vi "Message References to Message Handles.vi"(8 "error in":errorcluster, 11 "message refs":T2[](array[typedef]) format="%.0x") -> (0 "error out":errorcluster, 3 "message handles":cluster{"parameters":T1[], "timestamps":T2[]} {"timestamps" format="%.0x"; "parameters"."RxBC channel handle" format="%.0x"; "parameters"."RxRT channel handle" format="%.0x"; "parameters"."Tx channel handle" format="%.0x"})   [LabVIEW 2020, in "Ballard MIL-STD-1553 Engine.lvlib" / "Implementation.lvlib" / "Execution Unit.lvclass"]
uses:
  Execution Unit.lvclass
  <vilib>/NI VeriStand/Custom Device API/Custom Device Item Ref.ctl
  <vilib>/NI VeriStand/Custom Device API/Custom Device API.lvlib
  Scripting/Ballard MIL-STD-1553 Scripting.lvlib
  Parameter Handles.ctl
  Message Handles.ctl
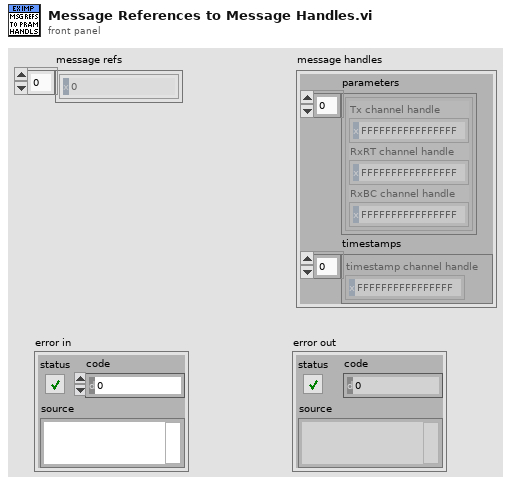
[diagram p1: front panel]
types:
  T1 = typedef "Ballard MIL-STD-1553 Engine.lvlib/Implementation.lvlib/Execution Unit.lvclass/Parameter Handles.ctl" = cluster{"Tx channel handle":T2, "RxRT channel handle":T2, "RxBC channel handle":T2}
  T2 = typedef "Custom Device API.lvlib/Custom Device Item Ref.ctl" = u64
  T3 = typedef "Ballard MIL-STD-1553 Engine.lvlib/Implementation.lvlib/Execution Unit.lvclass/Message Handles.ctl" = cluster{"parameters":T1[], "timestamps":T2[]}
  T4 = typedef "Direction.ctl" = enum16{"Rx", "Tx"}
  T5 = typedef "Terminal Endpoint.ctl" = cluster{"terminal address":T6, "subaddress":T6}
  T6 = typedef "Address.ctl" = u16
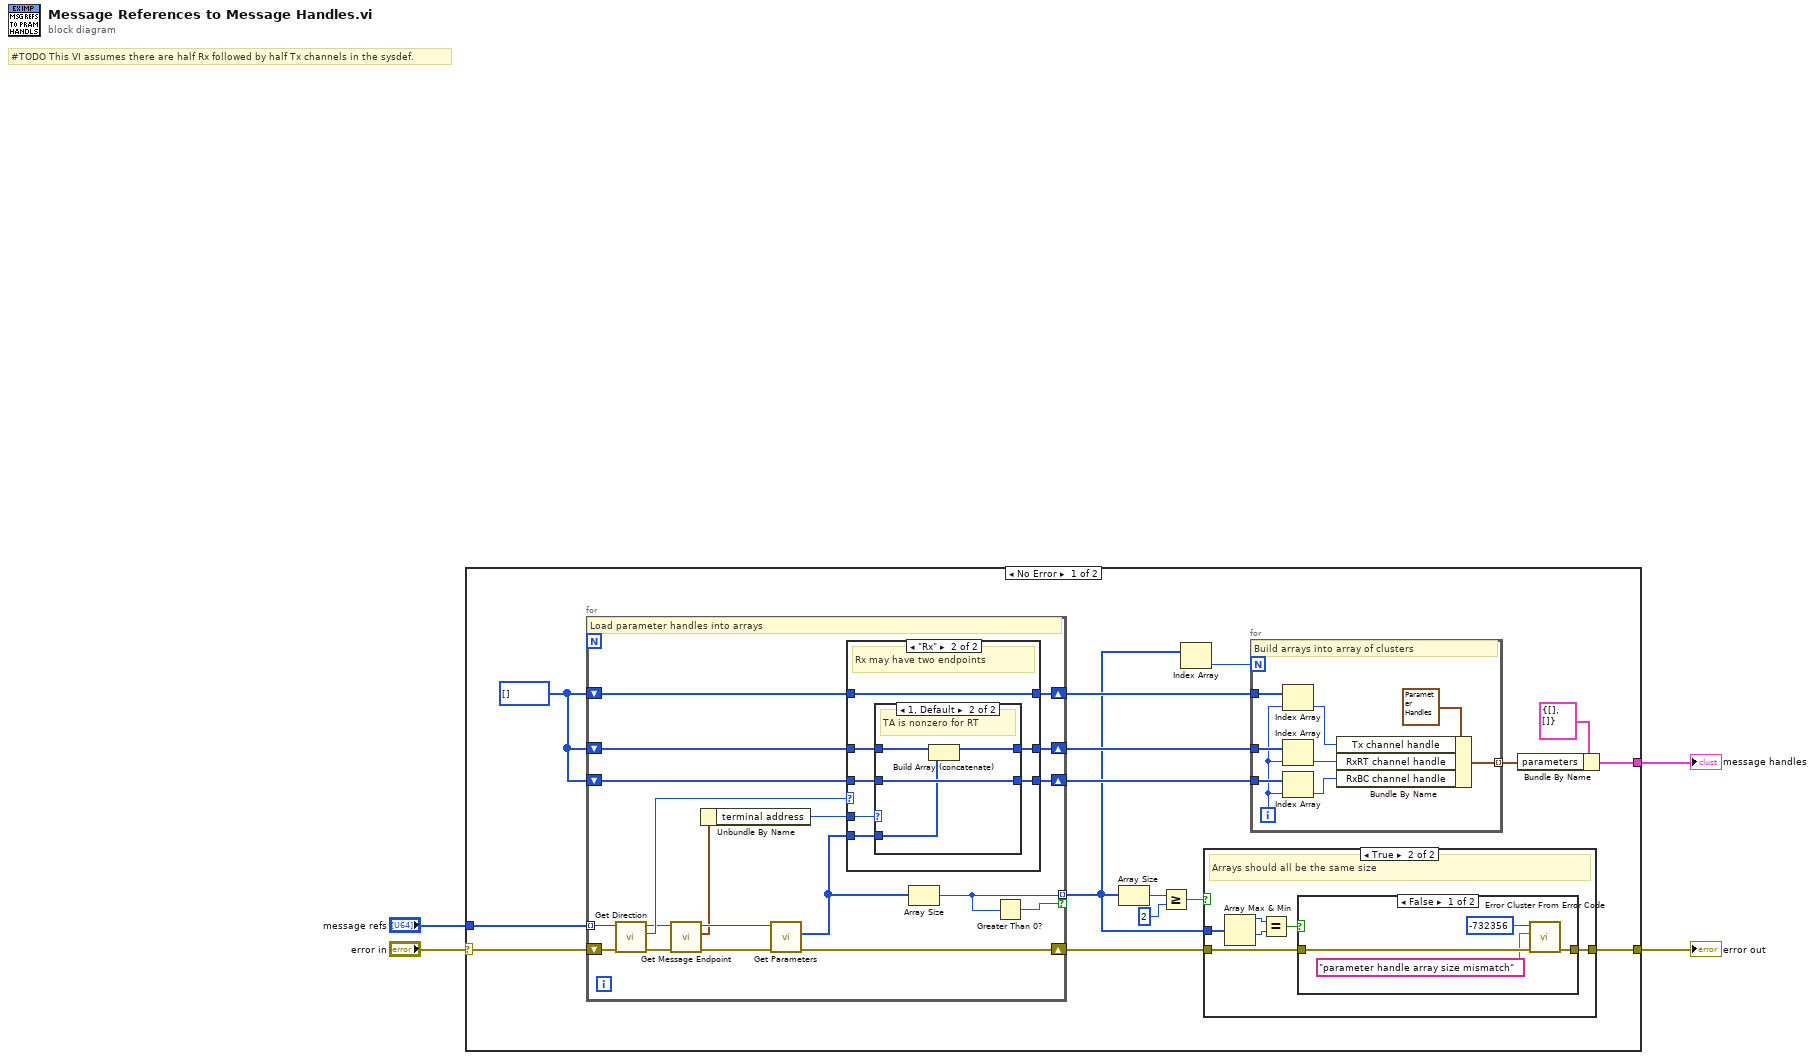
[diagram p0: block diagram]
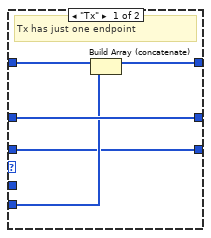
[diagram p4: hidden frame]
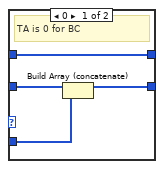
[diagram p5: hidden frame]
diagram:
  # "#TODO This VI assumes there are half Rx followed by half Tx channels in the sysdef."
  n1 = case shown="No Error" "error in" {
    selector: "error in" -> [w8 w81]
    tunnel: [w20 w81] -> w3
    tunnel: "message refs" -> [w7 _]
    tunnel: [w6 _] -> w1
    frame No Error {
      w19 = T2[] [] ("parameters")
      n2 = for {
        shift-right: [w54] -> w9
        shift-left: w8 -> [w53]
        tunnel: w7 -> [w52] mode=indexing
        shift-right: [w55] -> w15
        shift-left: w19 -> [w60]
        shift-right: [w56] -> w14
        shift-left: w19 -> [w59]
        shift-right: [w57] -> w16
        shift-left: w19 -> [w58]
        tunnel: [w42] -> w10 mode=indexing if=w43
        # "Load parameter handles into arrays"
        n3 = call "Get Direction.vi"("error in"=w53, "message in"=w52) -> ("error out"=w48:errorcluster, "direction"=w51:T4, "message out"=w50:T2)  [unwired: 6 in, 1 out]
        n4 = call "Get Message Endpoint.vi"("error in"=w48, "message in"=w50) -> ("error out"=w47:errorcluster, "message endpoint"=w46:T5, "message out"=w49:T2)  [unwired: 7 in]
        n5 = Unbundle By Name(w46) -> ("terminal address"=w45:T6)
        n6 = call "Get Parameters.vi"("error in"=w47, "message in"=w49) -> ("error out"=w54:errorcluster, "parameters"=w44:T2[])  [unwired: 7 in, 1 out]
        n7 = case shown="\"Rx\"" w51 {
          tunnel: w44 -> [w62 w66]
          tunnel: w60 -> [w61 w70]
          tunnel: w59 -> [w65 w68]
          tunnel: w58 -> [w64 w71]
          tunnel: [w63 w71] -> w57
          tunnel: [w65 w67] -> w56
          tunnel: [w61 w69] -> w55
          tunnel: w45 -> [_ w72]
          frame "Tx" {
            # "Tx has just one endpoint"
            n8 = Build Array (concatenate)(w64, w62) -> (w63:T2[])
          }
          frame "Rx" {
            # "Rx may have two endpoints"
            n9 = case shown="1, Default" w72 {
              tunnel: w70 -> [w76 w80]
              tunnel: [w75 w80] -> w69
              tunnel: w68 -> [w73 w79]
              tunnel: [w73 w78] -> w67
              tunnel: w66 -> [w74 w77]
              frame 0 {
                # "TA is 0 for BC"
                n10 = Build Array (concatenate)(w76, w74) -> (w75:T2[])
              }
              frame 1, Default {
                # "TA is nonzero for RT"
                n11 = Build Array (concatenate)(w79, w77) -> (w78:T2[])
              }
            }
          }
        }
        n12 = Array Size(array=w44) -> (size(s)=w42:i32)
        n13 = Greater Than 0?(x=w42) -> (x > 0?=w43:bool)
      }
      n14 = Array Size(array=w10) -> (size(s)=w13:i32)
      n15 = Greater Or Equal?(x=w13, y=2) -> (x >= y?=w11:bool)
      n16 = Index Array(array=w10) -> (element=w17:i32)  [unwired: 1 in]
      n17 = case shown="True" w11 {
        tunnel: w10 -> [_ w27]
        tunnel: w9 -> [w21 w22]
        tunnel: [w21 w24] -> w20
        frame False {
        }
        frame True {
          # "Arrays should all be the same size"
          n18 = Array Max & Min(array=w27) -> (max value=w25:i32, min value=w26:i32)  [unwired: 2 out]
          n19 = Equal?(x=w25, y=w26) -> (x = y?=w23:bool)
          n20 = case shown="False" w23 {
            tunnel: [w31 w32] -> w24
            tunnel: w22 -> [w29 w32]
            frame False {
              n21 = call <vilib>:"Error Cluster From Error Code.vi"("error in (no error)"=w29, "error message (\"\")"="parameter handle array size mismatch" ("format string"), "error code (0)"=-732356) -> ("error out"=w31:errorcluster)  [unwired: 6 in]
            }
            frame True {
            }
          }
        }
      }
      n22 = for {
        N: w17 -> [_]
        tunnel: w16 -> [w41]
        tunnel: w14 -> [w40]
        tunnel: w15 -> [w39]
        tunnel: [w35] -> w18 mode=indexing
        i -> [w34]
        # "Build arrays into array of clusters"
        n23 = Index Array(array=w41, index=w34) -> (element=w38:T2)
        n24 = Index Array(array=w40, index=w34) -> (element=w37:T2)
        n25 = Index Array(array=w39, index=w34) -> (element=w36:T2)
        n26 = Bundle By Name(cluster=T1 {"Tx channel handle"=18446744073709551615, "RxRT channel handle"=18446744073709551615, "RxBC channel handle"=18446744073709551615} ("parameter handles"), "Tx channel handle"=w38, "RxRT channel handle"=w37, "RxBC channel handle"=w36) -> (w35:T1)
      }
      n27 = Bundle By Name(cluster=T3 {"parameters"=[], "timestamps"=[]} ("message handles"), "parameters"=w18) -> (w6:T3)
    }
    frame Error {
    }
  }
  "error out" <- w3
  "message handles" <- w1
